vi "Main Application.vi"() -> ()   [LabVIEW 2024]
panel:
  in  "Enum":enum16{"read", "write"}(ring)
  out "Array":u16[](array[ring]) items=["Austin, TX", "New York City, NY", "Chicago, IL"]
  out "Gender":enum32{"Male", "Female"}[](array[ring])
  out "Info":string[](array[string])
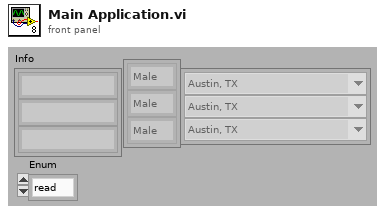
[diagram p1: front panel]
types:
  T1 = enum16{"open", "replace", "create", "open or create", "replace or create", "replace or create with confirmation"}
  T2 = cluster{"Name":string, "Gender":enum32{"Radio Selection 1", "Radio Selection 2"}, "Location":u16}
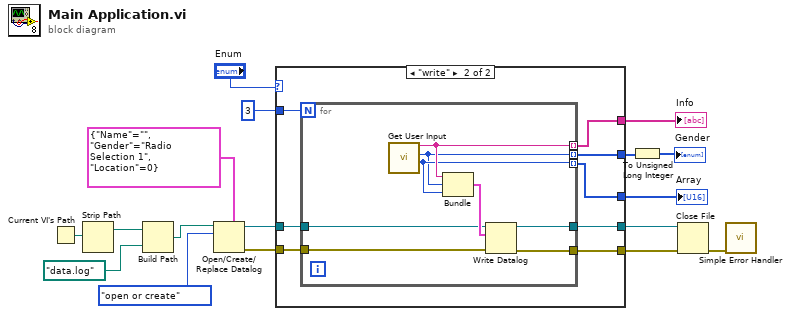
[diagram p0: block diagram]
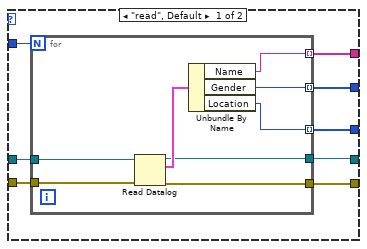
[diagram p2: hidden frame]
diagram:
  n1 = Current VI's Path() -> (path=w3:path)
  n2 = Strip Path(path=w3) -> (stripped path=w2:path)  [unwired: 1 out]
  n3 = Build Path(base path=w2, name or relative path=path "data.log" ("datalog path (use dialog)")) -> (appended path=w4:path)
  n4 = Open/Create/Replace Datalog(5:T2 {"Name"="", "Gender"=enum."Radio Selection 1", "Location"=0} ("output cluster"), 10:T1."open or create" ("operation (0:open)"), 11:w4) -> (0:w12:errorcluster, 3:w15:refnum<k1>)  [unwired: 1 in, 3 out]
  n5 = case shown="\"write\"" "Enum" {
    tunnel: [w22 w41] -> w17
    tunnel: [w21 w34] -> w7
    tunnel: [w20 w40] -> w16
    tunnel: w15 -> [w24 w39]
    tunnel: [w19 w38] -> w13
    tunnel: w12 -> [w23 w37]
    tunnel: [w18 w36] -> w11
    tunnel: 3 -> [w25 w35]
    frame "read", Default {
      n6 = for {
        N: w25 -> [_]
        tunnel: w24 -> [w33]
        tunnel: w23 -> [w32]
        tunnel: [w30] -> w22 mode=indexing
        tunnel: [w29] -> w21 mode=indexing
        tunnel: [w28] -> w20 mode=indexing
        tunnel: [w27] -> w19
        tunnel: [w26] -> w18
        n7 = Read Datalog(4:w32, 7:w33) -> (0:w26:errorcluster, 2:w31:T2, 3:w27:refnum<k1>)  [unwired: 1 out]
        n8 = Unbundle By Name(w31) -> ("Name"=w30:string, "Gender"=w29:enum32{"Radio Selection 1", "Radio Selection 2"}, "Location"=w28:u16)
      }
    }
    frame "write" {
      n9 = for {
        N: w35 -> [_]
        tunnel: [w49] -> w41 mode=indexing
        tunnel: [w47] -> w34 mode=indexing
        tunnel: [w48] -> w40 mode=indexing
        tunnel: w39 -> [w45]
        tunnel: [w44] -> w38
        tunnel: w37 -> [w43]
        tunnel: [w42] -> w36
        n10 = call "Get User Input.vi"() -> ("Location"=w48:u16, "Gender"=w47:enum32{"Radio Selection 1", "Radio Selection 2"}, "Name"=w49:string)  [unwired: 3 in, 6 out]
        n11 = Bundle("Name"=w49, "Gender"=w47, "Location"=w48) -> (w46:T2)  [unwired: 1 out]
        n12 = Write Datalog(4:w43, 6:w46, 7:w45) -> (0:w42:errorcluster, 3:w44:refnum<k1>)
      }
    }
  }
  "Info" <- w17
  "Array" <- w16
  n13 = To Unsigned Long Integer(number=w7) -> (unsigned 32bit integer=→"Gender":u32[])
  n14 = Close File(refnum=w13, error in=w11) -> (error out=w1:errorcluster)  [unwired: 1 out]
  n15 = call <vilib>:"Simple Error Handler.vi"("error in (no error)"=w1) -> ()  [unwired: 1 in, 8 out]
